vi "H5Pset_multi_type.vi"(6 "error in (no error)":errorcluster, 8 "Member Type":T1 items=["H5FD_MEM_NOLIST"=-1, "H5FD_MEM_DEFAULT"=0, "H5FD_MEM_SUPER"=1, "H5FD_MEM_BTREE"=2, "H5FD_MEM_DRAW"=3, "H5FD_MEM_GHEAP"=4, "H5FD_MEM_LHEAP"=5, "H5FD_MEM_OHDR"=6], 9 "HDF5 Property List Ref":T2) -> (0 "error out":errorcluster, 3 "HDF5 Property List Ref out":T2)   [LabVIEW 2017]
doc: "Specifies type of data to be accessed via the MULTI driver, \n enabling more direct access."
uses:
  <vilib>/UPVI/lvhdf5/library.llb/HDF5 Ref.ctl
  <vilib>/UPVI/lvhdf5/property.llb/H5FD_mem_t.ctl
  <vilib>/UPVI/lvhdf5/hdf5.dll
panel:
  # "LVHDF5 Toolkit\nCopyright (c) 2005-2013 by Jason D. Sommerville\nCopyright (c) 2014 by UPVI, LLC.\n\nThis use and distribution of this file is governed by the terms found in \nLICENSE.txt distributed with this toolkit and installed at\n <user.lib>\\_lvhdf5\\LICENSE.txt"
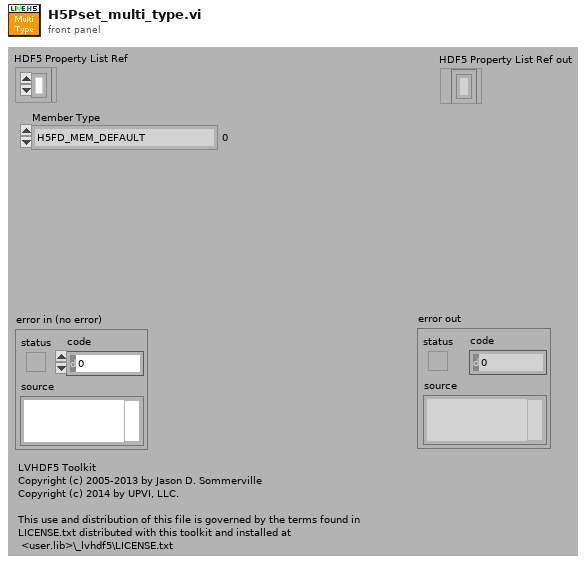
[diagram p1: front panel]
types:
  T1 = typedef "H5FD_mem_t.ctl" = i32
  T2 = typedef "HDF5 Ref.ctl" = refnum<k1>
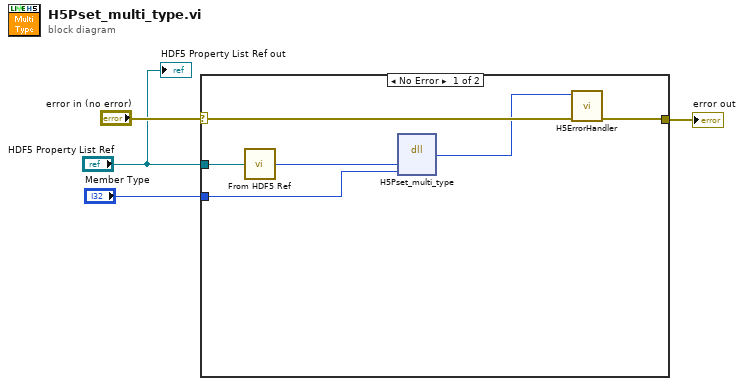
[diagram p0: block diagram]
diagram:
  n1 = case shown="No Error" "error in (no error)" {
    selector: "error in (no error)" -> [w10 w11]
    tunnel: [w9 w11] -> w3
    tunnel: "HDF5 Property List Ref" -> [w8 _]
    tunnel: "Member Type" -> [w5 _]
    frame No Error {
      n2 = call <vilib>:"From HDF5 Ref.vi"("HDF5 Ref"=w8) -> ("I32"=w7:i32)
      n3 = dll-call lib="C:/Program Files/National Instruments/LabVIEW 2017/vi.lib/UPVI/lvhdf5/hdf5.dll" fn="H5Pset_multi_type"("plist_id"=w7, "type"=w5) -> (w6:i32)  [unwired: 5 in, 2 out]
      n4 = call <vilib>:"H5ErrorHandler.vi"("error in (no error)"=w10, "herr_t"=w6) -> ("error out"=w9:errorcluster)  [unwired: 3 in, 4 out]
    }
    frame Error {
    }
  }
  "error out" <- w3
  "HDF5 Property List Ref out" <- "HDF5 Property List Ref"
